vi "间隙计算.vi"(10 "扭矩数组":dbl[](array[numeric])) -> (0 "扭差":dbl format="%#.2f", 1 "平均扭矩":dbl format="%#.2f", 2 "最小扭矩":dbl, 3 "峰值间隙1":dbl format="%#.2f", 4 "峰值间隙2":dbl format="%#.2f")   [LabVIEW 2013]
panel:
  out "第一个子数组":dbl[](array[numeric])
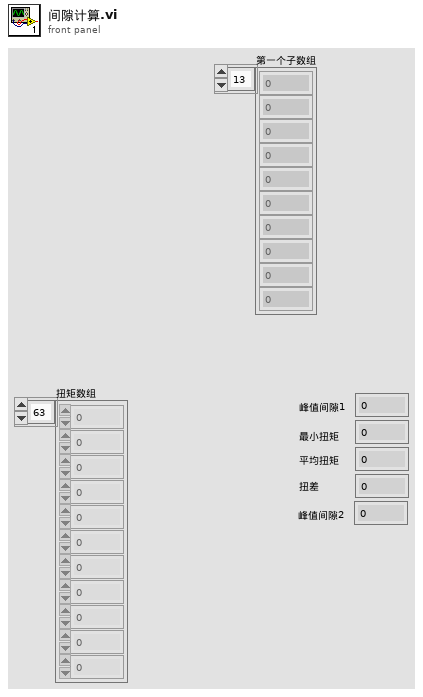
[diagram p1: front panel]
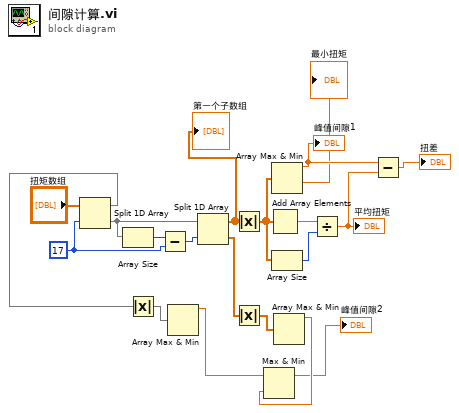
[diagram p0: block diagram]
diagram:
  w10 = 17 ("索引")
  n1 = Split 1D Array(array="扭矩数组", index=w10) -> (first subarray=w7:dbl[], second subarray=w12:dbl[])
  n2 = Array Size(array=w12) -> (size(s)=w11:i32)
  n3 = Absolute Value(x=w7) -> (abs(x)=w6:dbl[])
  n4 = Subtract(x=w11, y=w10) -> (x-y=w9:i32)
  n5 = Array Max & Min(array=w6) -> (max value=w3:dbl)  [unwired: 3 out]
  n6 = Split 1D Array(array=w12, index=w9) -> (first subarray=w16:dbl[], second subarray=w5:dbl[])
  "第一个子数组" <- w16
  n7 = Absolute Value(x=w16) -> (abs(x)=w18:dbl[])
  n8 = Absolute Value(x=w5) -> (abs(x)=w4:dbl[])
  n9 = Add Array Elements(numeric array=w18) -> (sum=w19:dbl)
  n10 = Array Max & Min(array=w18) -> (max value=w15:dbl, min value=→"最小扭矩":dbl)  [unwired: 2 out]
  "峰值间隙1" <- w15
  n11 = Array Size(array=w18) -> (size(s)=w17:i32)
  n12 = Array Max & Min(array=w4) -> (max value=w2:dbl)  [unwired: 3 out]
  n13 = Max & Min(x=w3, y=w2) -> (max(x,y)=→"峰值间隙2":dbl)  [unwired: 1 out]
  n14 = Divide(x=w19, y=w17) -> (x/y=w14:dbl)
  "平均扭矩" <- w14
  n15 = Subtract(x=w15, y=w14) -> (x-y=→"扭差":dbl)
